vi "5302GetPhaseVISA.vi"(8 "error in (no error)":errorcluster, 11 "VISA session (for class)":refnum<visa-resource-name>) -> (0 "error out":errorcluster, 1 "data string":string, 2 "Phase":dbl format="%.4f", 3 "VISA session":refnum<visa-resource-name>)   [LabVIEW 2015]
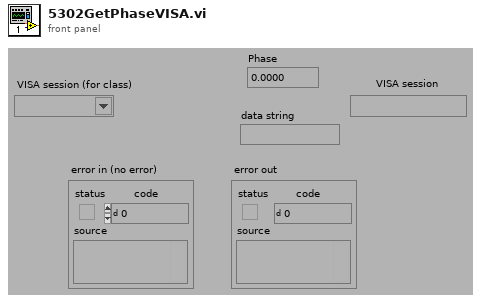
[diagram p1: front panel]
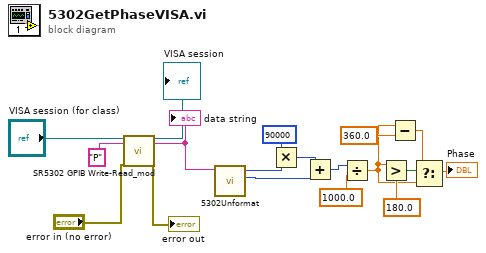
[diagram p0: block diagram]
diagram:
  n1 = call "SR5302 GPIB Write-Read_mod.vi"("VISA session (for class)"="VISA session (for class)", "Write Command String"="P" ("data string"), "error in (no error)"="error in (no error)") -> ("VISA session"=→"VISA session":refnum<visa-resource-name>, "Response 1"=w1:string, "error out"=→"error out":errorcluster)  [unwired: 5 in, 9 out]
  "data string" <- w1
  n2 = call "5302Unformat.vi"("Data String"=w1) -> ("Numeric 2"=w4:i32, "Numeric 1"=w5:i32)  [unwired: 9 in]
  n3 = Multiply(x=90000 ("y"), y=w5) -> (x*y=w13:i32)
  n4 = Add(x=w13, y=w4) -> (x+y=w15:i32)
  n5 = Divide(x=w15, y=1000.0) -> (x/y=w7:dbl)
  n6 = Greater?(x=w7, y=180.0) -> (0:w10:bool)
  n7 = Subtract(x=w7, y=360.0) -> (x-y=w8:dbl)
  n8 = Select(t=w8, s=w10, f=w7) -> (s? t:f=→"Phase":dbl)
